vi "1B.3-Spoof Relative Wind.vi"(3 "Wind Speed":dbl, 4 "Wind Angle":T1 format="%05.1f", 5 "Velocity (3 array)":dbl[](array[numeric])) -> (0 "Perceived Wind":cluster{"X Position":dbl, "Y Position":dbl}, 1 "Global Wind":cluster{"X Position":dbl, "Y Position":dbl}, 2 "Orientation":cluster{"X Position":dbl, "Y Position":dbl})   [LabVIEW 2011]
uses:
  2-RIO/2 Typedefs/heading.ctl
  <vilib>/Analysis/_algsub.llb/Real Vector Norm.vi
  <vilib>/Analysis/baseanly.llb/Real Dot Product.vi
  <vilib>/Analysis/NI_AALPro.lvlib
  <vilib>/Analysis/NI_AALBase.lvlib
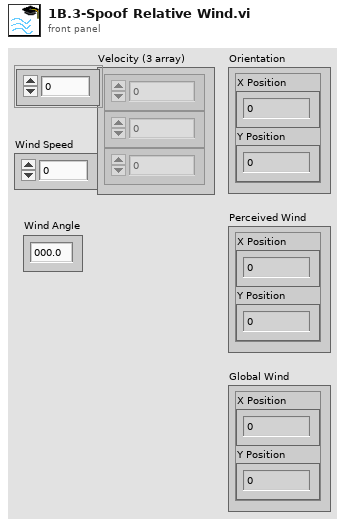
[diagram p1: front panel]
types:
  T1 = typedef "heading.ctl" = dbl
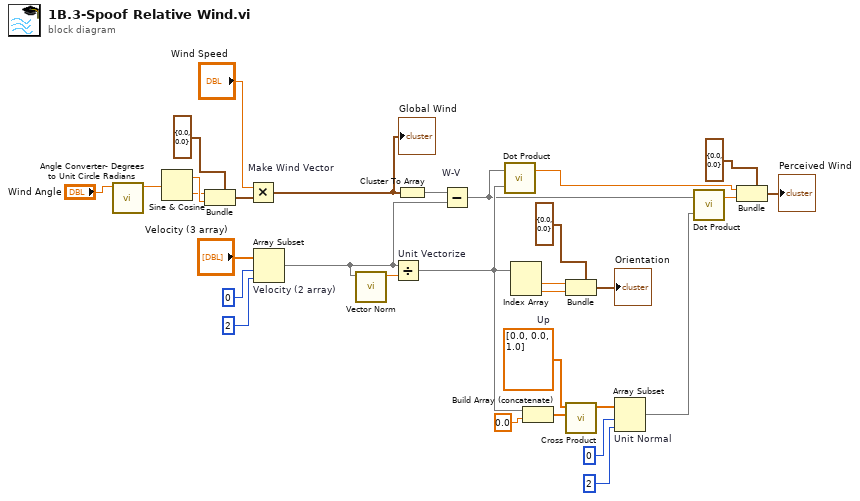
[diagram p0: block diagram]
diagram:
  w3 = dbl[] [0.0, 0.0, 1.0]  # Up
  n1 = call "Angle Converter- Degrees to Unit Circle Radians.vi"("Angle in \nHeading \nFormat"="Wind Angle") -> ("Angle in \nUnit Circle\nRadians"=w2:dbl)  [unwired: 10 in]
  n2 = Sine & Cosine(0:w2) -> (1:w18:dbl, 2:w17:dbl)
  n3 = Bundle(cluster=cluster{"X Position":dbl, "Y Position":dbl} {"X Position"=0.0, "Y Position"=0.0} ("Robot Location"), "X Position"=w17, "Y Position"=w18) -> (w19:cluster{"X Position":dbl, "Y Position":dbl})
  n4 = Multiply "Make Wind Vector"(x="Wind Speed", y=w19) -> (x*y=w22:cluster{"X Position":dbl, "Y Position":dbl})
  "Global Wind" <- w22
  n5 = Array Subset "Velocity (2 array)"(array="Velocity (3 array)", index=0, length=2) -> (w13:dbl[])
  n6 = call-poly <vilib>:"Vector Norm.vi"("Input Vector"=w13) -> ("norm"=w31:dbl)  [unwired: 9 in, 1 out]
  n7 = Divide "Unit Vectorize"(x=w13, y=w31) -> (x/y=w12:dbl[])
  n8 = Cluster To Array(cluster=w22) -> (array=w27:dbl[])
  n9 = Subtract "W-V"(x=w27, y=w13) -> (x-y=w7:dbl[])
  n10 = call-poly <vilib>:"Dot Product.vi"("Y Vector"=w12, "X Vector"=w7) -> ("X * Y"=w29:dbl)  [unwired: 1 out]
  n11 = Index Array(array=w12) -> (element #1=w24:dbl, element #2=w25:dbl)  [unwired: 2 in]
  n12 = Build Array (concatenate)(w12, 0.0) -> (w4:dbl[])
  n13 = Bundle(cluster=cluster{"X Position":dbl, "Y Position":dbl} {"X Position"=0.0, "Y Position"=0.0} ("Robot Location"), "X Position"=w24, "Y Position"=w25) -> (→"Orientation":cluster{"X Position":dbl, "Y Position":dbl})
  n14 = call <vilib>:"Cross Product.vi"("B Vector"=w4, "A Vector"=w3) -> ("Cross Product"=w8:dbl[])  [unwired: 8 in, 1 out]
  n15 = Array Subset "Unit Normal"(array=w8, index=0, length=2) -> (w6:dbl[])
  n16 = call-poly <vilib>:"Dot Product.vi"("Y Vector"=w6, "X Vector"=w7) -> ("X * Y"=w5:dbl)  [unwired: 1 out]
  n17 = Bundle(cluster=cluster{"X Position":dbl, "Y Position":dbl} {"X Position"=0.0, "Y Position"=0.0} ("Perceived Wind"), "X Position"=w29, "Y Position"=w5) -> (→"Perceived Wind":cluster{"X Position":dbl, "Y Position":dbl})
